vi "Assert True.vi"(8 "error in":errorcluster, 10 "failure message":string, 11 "condition":bool) -> (0 "error out":errorcluster, 2 "message":string, 3 "pass":bool)   [LabVIEW 2021, in "MeasurementServerTests.lvlib"]
uses:
  MeasurementServerTests.lvlib
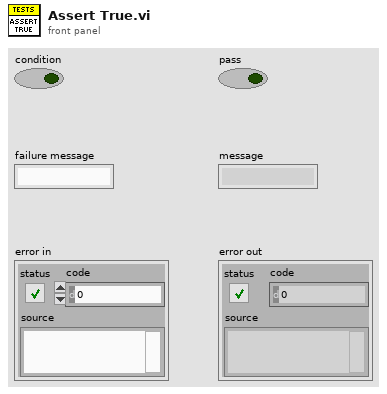
[diagram p1: front panel]
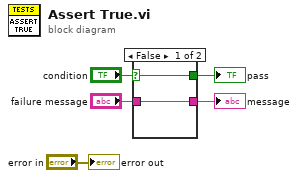
[diagram p0: block diagram]
diagram:
  n1 = case shown="False" "condition" {
    selector: "condition" -> [w7 w8]
    tunnel: [w7 w8] -> w3
    tunnel: "failure message" -> [w6 _]
    tunnel: [w6 _] -> w1
    frame False {
    }
    frame True {
    }
  }
  "message" <- w1
  "pass" <- w3
  "error out" <- "error in"
